vi "Page Sixe points.vi"() -> ()   [LabVIEW 2019]
uses:
  <userlib>/Exaprom PDF/Controls/Page Controls/Page size.ctl
  <userlib>/Exaprom PDF/Controls/Page Controls/Page Orientation.ctl
  C:/Program Files/National Instruments/LabVIEW 2019/user.lib/Exaprom PDF/DLL/itextsharp.dll
  DLL/itextsharp.dll
panel:
  out "Resulting page":T2
  in  "Page Size":cluster{"Width":sgl, "Height":sgl}
  in  "Orientation":T1
  out "Landscape":T3(array[cluster])
  out "Portrait":T3(array[cluster])
  out "Array":T4(array[cluster])
  in  "Page Size":T5=10 items=["Custom", "LETTER", "NOTE", "LEGAL", "TABLOID", "EXECUTIVE", "POSTCARD", "A0", "A1", "A2", "A3", "A4", "A5", "A6", "A7", "A8", "A9", "A10", "B0", "B1", "B2", "B3", "B4", "B5", "B6", "B7", "B8", "B9", "B10", "ARCH_E", "ARCH_D", "ARCH_C", "ARCH_B", "ARCH_A", "FLSA", "FLSE", "HALFLETTER", "_11X17", "ID_1", "ID_2", "ID_3", "LEDGER", "CROWN_QUARTO", "LARGE_CROWN_QUARTO", "DEMY_QUARTO", "ROYAL_QUARTO", "CROWN_OCTAVO", "LARGE_CROWN_OCTAVO", "DEMY_OCTAVO", "ROYAL_OCTAVO", "SMALL_PAPERBACK", "PENGUIN_SMALL_PAPERBACK", "PENGUIN_LARGE_PAPERBACK"]
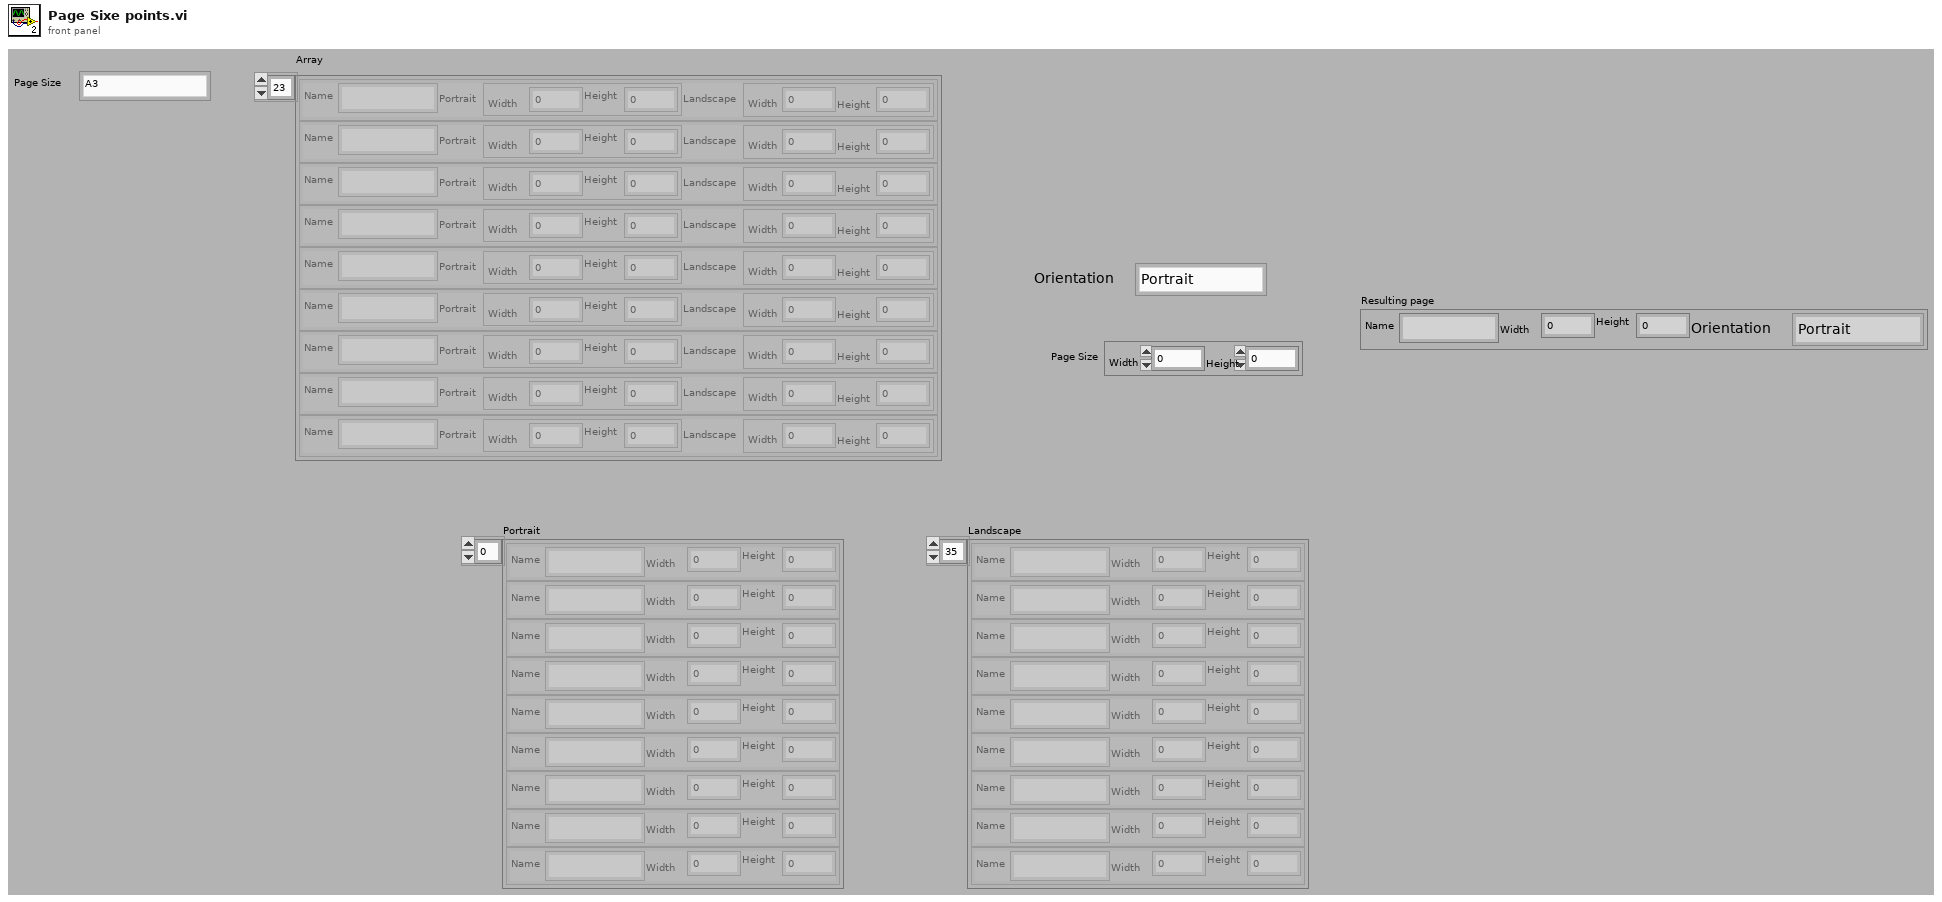
[diagram p1: front panel]
types:
  T1 = typedef "Page Orientation.ctl" = enum16{"Portrait", "Landscape"}
  T2 = cluster{"Name":string, "Width":sgl, "Height":sgl, "Orientation":T1}
  T3 = cluster{"Name":string, "Width":sgl, "Height":sgl}[]
  T4 = cluster{"Name":string, "Portrait":cluster{"Width":sgl, "Height":sgl}, "Landscape":cluster{"Width":sgl, "Height":sgl}}[]
  T5 = typedef "Page size.ctl" = i32
  T6 = cluster{string, cluster{"Width":sgl, "Height":sgl}, cluster{"Width":sgl, "Height":sgl}}
  T7 = cluster{"f":string, "Width":sgl, "Height":sgl, "Orientation":T1}
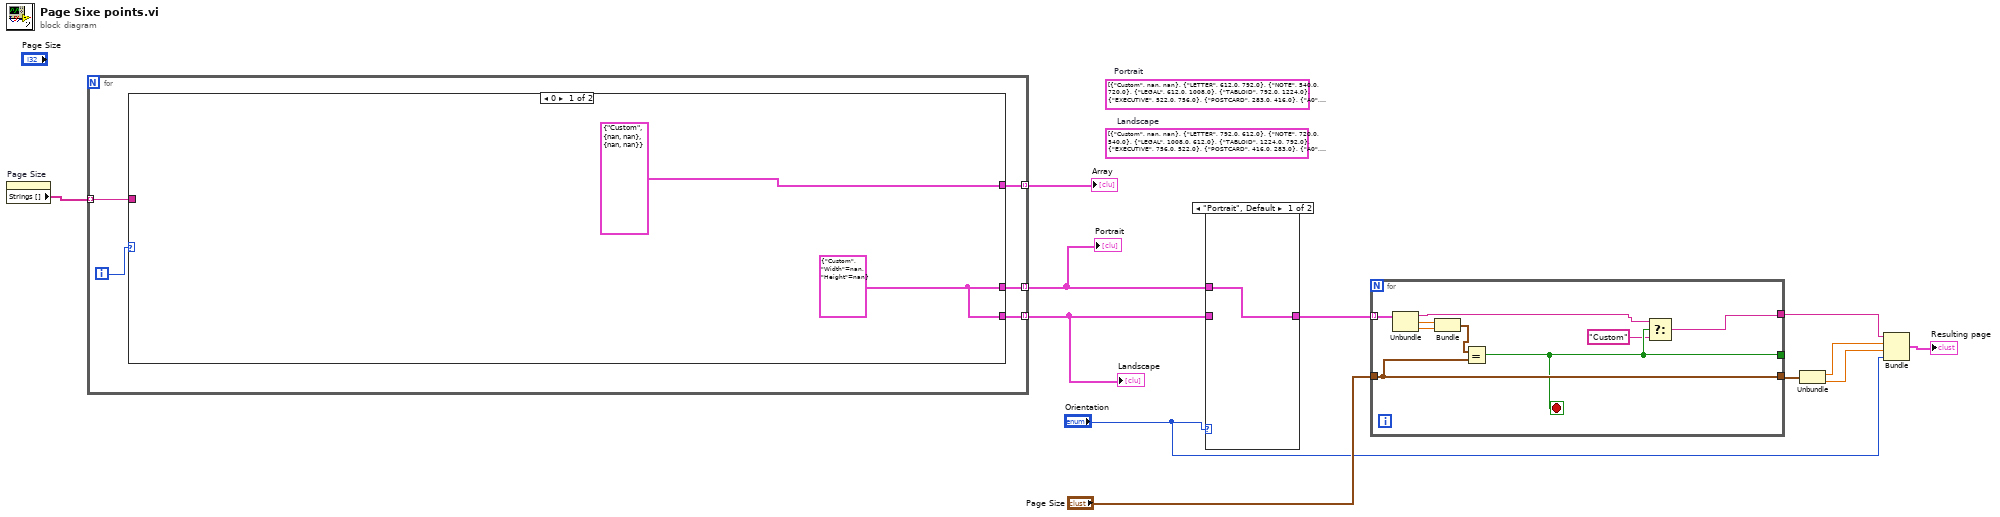
[diagram p0: block diagram]
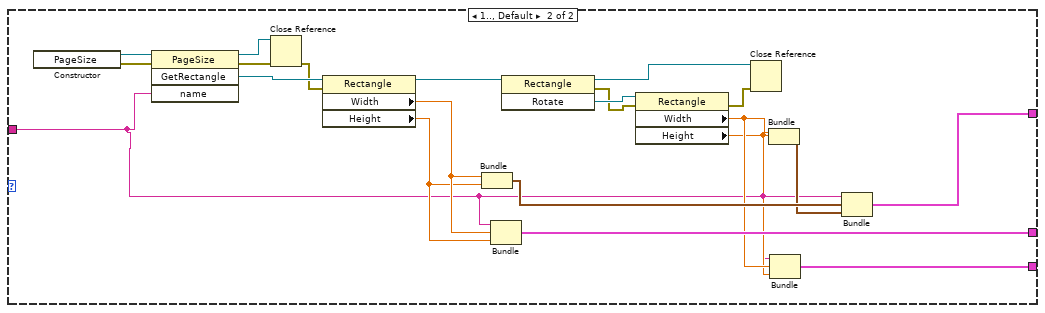
[diagram p3: hidden frame]
diagram:
  (unwired) T3 [{"Name"="Custom", "Width"=nan, "Height"=nan}, {"Name"="LETTER", "Width"=792.0, "Height"=612.0}, {"Name"="NOTE", "Width"=720.0, "Height"=540.0}, {"Name"="LEGAL", "Width"=1008.0, "Height"=612.0}, {"Name"="TABLOID", "Width"=1224.0, "Height"=792.0}, {"Name"="EXECUTIVE", "Width"=756.0, "Height"=522.0}, {"Name"="POSTCARD", "Width"=416.0, "Height"=283.0}, {"Name"="A0", "Width"=3370.0, "Height"=2384.0}, {"Name"="A1", "Width"=2384.0, "Height"=1684.0}, {"Name"="A2", "Width"=1684.0, "Height"=1191.0}, {"Name"="A3", "Width"=1191.0, "Height"=842.0}, {"Name"="A4", "Width"=842.0, "Height"=595.0}, {"Name"="A5", "Width"=595.0, "Height"=420.0}, {"Name"="A6", "Width"=420.0, "Height"=297.0}, {"Name"="A7", "Width"=297.0, "Height"=210.0}, {"Name"="A8", "Width"=210.0, "Height"=148.0}, {"Name"="A9", "Width"=148.0, "Height"=105.0}, {"Name"="A10", "Width"=105.0, "Height"=73.0}, {"Name"="B0", "Width"=4008.0, "Height"=2834.0}, {"Name"="B1", "Width"=2834.0, "Height"=2004.0}, {"Name"="B2", "Width"=2004.0, "Height"=1417.0}, {"Name"="B3", "Width"=1417.0, "Height"=1000.0}, {"Name"="B4", "Width"=1000.0, "Height"=708.0}, {"Name"="B5", "Width"=708.0, "Height"=498.0}, {"Name"="B6", "Width"=498.0, "Height"=354.0}, {"Name"="B7", "Width"=354.0, "Height"=249.0}, {"Name"="B8", "Width"=249.0, "Height"=175.0}, {"Name"="B9", "Width"=175.0, "Height"=124.0}, {"Name"="B10", "Width"=124.0, "Height"=87.0}, {"Name"="ARCH_E", "Width"=3456.0, "Height"=2592.0}, {"Name"="ARCH_D", "Width"=2592.0, "Height"=1728.0}, {"Name"="ARCH_C", "Width"=1728.0, "Height"=1296.0}, {"Name"="ARCH_B", "Width"=1296.0, "Height"=864.0}, {"Name"="ARCH_A", "Width"=864.0, "Height"=648.0}, {"Name"="FLSA", "Width"=936.0, "Height"=612.0}, {"Name"="FLSE", "Width"=936.0, "Height"=648.0}, {"Name"="HALFLETTER", "Width"=612.0, "Height"=396.0}, {"Name"="_11X17", "Width"=1224.0, "Height"=792.0}, {"Name"="ID_1", "Width"=153.0, "Height"=242.65}, {"Name"="ID_2", "Width"=210.0, "Height"=297.0}, {"Name"="ID_3", "Width"=249.0, "Height"=354.0}, {"Name"="LEDGER", "Width"=792.0, "Height"=1224.0}, {"Name"="CROWN_QUARTO", "Width"=697.0, "Height"=535.0}, {"Name"="LARGE_CROWN_QUARTO", "Width"=731.0, "Height"=569.0}, {"Name"="DEMY_QUARTO", "Width"=782.0, "Height"=620.0}, {"Name"="ROYAL_QUARTO", "Width"=884.0, "Height"=671.0}, {"Name"="CROWN_OCTAVO", "Width"=527.0, "Height"=348.0}, {"Name"="LARGE_CROWN_OCTAVO", "Width"=561.0, "Height"=365.0}, {"Name"="DEMY_OCTAVO", "Width"=612.0, "Height"=391.0}, {"Name"="ROYAL_OCTAVO", "Width"=663.0, "Height"=442.0}, {"Name"="SMALL_PAPERBACK", "Width"=504.0, "Height"=314.0}, {"Name"="PENGUIN_SMALL_PAPERBACK", "Width"=513.0, "Height"=314.0}, {"Name"="PENGUIN_LARGE_PAPERBACK", "Width"=561.0, "Height"=365.0}]  # Landscape
  (unwired) T3 [{"Name"="Custom", "Width"=nan, "Height"=nan}, {"Name"="LETTER", "Width"=612.0, "Height"=792.0}, {"Name"="NOTE", "Width"=540.0, "Height"=720.0}, {"Name"="LEGAL", "Width"=612.0, "Height"=1008.0}, {"Name"="TABLOID", "Width"=792.0, "Height"=1224.0}, {"Name"="EXECUTIVE", "Width"=522.0, "Height"=756.0}, {"Name"="POSTCARD", "Width"=283.0, "Height"=416.0}, {"Name"="A0", "Width"=2384.0, "Height"=3370.0}, {"Name"="A1", "Width"=1684.0, "Height"=2384.0}, {"Name"="A2", "Width"=1191.0, "Height"=1684.0}, {"Name"="A3", "Width"=842.0, "Height"=1191.0}, {"Name"="A4", "Width"=595.0, "Height"=842.0}, {"Name"="A5", "Width"=420.0, "Height"=595.0}, {"Name"="A6", "Width"=297.0, "Height"=420.0}, {"Name"="A7", "Width"=210.0, "Height"=297.0}, {"Name"="A8", "Width"=148.0, "Height"=210.0}, {"Name"="A9", "Width"=105.0, "Height"=148.0}, {"Name"="A10", "Width"=73.0, "Height"=105.0}, {"Name"="B0", "Width"=2834.0, "Height"=4008.0}, {"Name"="B1", "Width"=2004.0, "Height"=2834.0}, {"Name"="B2", "Width"=1417.0, "Height"=2004.0}, {"Name"="B3", "Width"=1000.0, "Height"=1417.0}, {"Name"="B4", "Width"=708.0, "Height"=1000.0}, {"Name"="B5", "Width"=498.0, "Height"=708.0}, {"Name"="B6", "Width"=354.0, "Height"=498.0}, {"Name"="B7", "Width"=249.0, "Height"=354.0}, {"Name"="B8", "Width"=175.0, "Height"=249.0}, {"Name"="B9", "Width"=124.0, "Height"=175.0}, {"Name"="B10", "Width"=87.0, "Height"=124.0}, {"Name"="ARCH_E", "Width"=2592.0, "Height"=3456.0}, {"Name"="ARCH_D", "Width"=1728.0, "Height"=2592.0}, {"Name"="ARCH_C", "Width"=1296.0, "Height"=1728.0}, {"Name"="ARCH_B", "Width"=864.0, "Height"=1296.0}, {"Name"="ARCH_A", "Width"=648.0, "Height"=864.0}, {"Name"="FLSA", "Width"=612.0, "Height"=936.0}, {"Name"="FLSE", "Width"=648.0, "Height"=936.0}, {"Name"="HALFLETTER", "Width"=396.0, "Height"=612.0}, {"Name"="_11X17", "Width"=792.0, "Height"=1224.0}, {"Name"="ID_1", "Width"=242.65, "Height"=153.0}, {"Name"="ID_2", "Width"=297.0, "Height"=210.0}, {"Name"="ID_3", "Width"=354.0, "Height"=249.0}, {"Name"="LEDGER", "Width"=1224.0, "Height"=792.0}, {"Name"="CROWN_QUARTO", "Width"=535.0, "Height"=697.0}, {"Name"="LARGE_CROWN_QUARTO", "Width"=569.0, "Height"=731.0}, {"Name"="DEMY_QUARTO", "Width"=620.0, "Height"=782.0}, {"Name"="ROYAL_QUARTO", "Width"=671.0, "Height"=884.0}, {"Name"="CROWN_OCTAVO", "Width"=348.0, "Height"=527.0}, {"Name"="LARGE_CROWN_OCTAVO", "Width"=365.0, "Height"=561.0}, {"Name"="DEMY_OCTAVO", "Width"=391.0, "Height"=612.0}, {"Name"="ROYAL_OCTAVO", "Width"=442.0, "Height"=663.0}, {"Name"="SMALL_PAPERBACK", "Width"=314.0, "Height"=504.0}, {"Name"="PENGUIN_SMALL_PAPERBACK", "Width"=314.0, "Height"=513.0}, {"Name"="PENGUIN_LARGE_PAPERBACK", "Width"=365.0, "Height"=561.0}]  # Portrait
  n1 = property on="Page Size" class="Ring (strict)"() -> ("Strings []"=w12:string[])  [unwired: 2 in, 2 out]
  n2 = for {
    tunnel: w12 -> [w17] mode=indexing
    tunnel: [w15] -> w11 mode=indexing
    tunnel: [w14] -> w9 mode=indexing
    tunnel: [w13] -> w10 mode=indexing
    i -> [w16]
    n3 = case shown="0" w16 {
      tunnel: w17 -> [_ w21]
      tunnel: [T6 {"Custom", {"Width"=nan, "Height"=nan}, {"Width"=nan, "Height"=nan}} w27] -> w15
      tunnel: [w18 w24] -> w14
      tunnel: [w18 w20] -> w13
      frame 0 {
        w18 = cluster{string, "Width":sgl, "Height":sgl} {"Custom", "Width"=nan, "Height"=nan}
      }
      frame 1.., Default {
        n4 = constructor class="PageSize"() -> (reference out=w40:refnum<k24>, error out=w39:errorcluster)  [unwired: 3 in, 1 out]
        n5 = invoke class="PageSize" method="GetRectangle"(reference=w40, error in=w39, "name"=w21) -> (reference out=w37:refnum<k24>, error out=w38:errorcluster, "GetRectangle"=w36:refnum<k24>)  [unwired: 1 in, 1 out]
        n6 = Close Reference(reference=w37, error in (no error)=w38) -> (error out=w35:errorcluster)
        n7 = property class="Rectangle"(reference=w36, error in=w35) -> (reference out=w33:refnum<k24>, "Width"=w26:sgl, "Height"=w25:sgl)  [unwired: 1 out]
        n8 = Bundle("Width"=w26, "Height"=w25) -> (w29:cluster{"Width":sgl, "Height":sgl})  [unwired: 1 in]
        n9 = Bundle(w21, "Width"=w26, "Height"=w25) -> (w24:cluster{string, "Width":sgl, "Height":sgl})  [unwired: 1 in]
        n10 = invoke class="Rectangle" method="Rotate"(reference=w33) -> (reference out=w34:refnum<k24>, error out=w30:errorcluster, "Rotate"=w31:refnum<k24>)  [unwired: 2 in]
        n11 = property class="Rectangle"(reference=w31, error in=w30) -> (error out=w32:errorcluster, "Width"=w23:sgl, "Height"=w22:sgl)  [unwired: 1 out]
        n12 = Close Reference(reference=w34, error in (no error)=w32) -> ()  [unwired: 1 out]
        n13 = Bundle("Width"=w23, "Height"=w22) -> (w28:cluster{"Width":sgl, "Height":sgl})  [unwired: 1 in]
        n14 = Bundle(w21, "Width"=w23, "Height"=w22) -> (w20:cluster{string, "Width":sgl, "Height":sgl})  [unwired: 1 in]
        n15 = Bundle(w21, w29, w28) -> (w27:T6)  [unwired: 1 in]
      }
    }
  }
  "Array" <- w11
  "Portrait" <- w9
  "Landscape" <- w10
  n16 = case shown="\"Portrait\", Default" "Orientation" {
    tunnel: [w41 w42] -> w8
    tunnel: w10 -> [_ w42]
    tunnel: w9 -> [w41 _]
    frame "Portrait", Default {
    }
    frame "Landscape" {
    }
  }
  n17 = for {
    tunnel: w8 -> [w51] mode=indexing
    tunnel: "Page Size" -> [w47]
    tunnel: [w43] -> w6
    tunnel: [w47] -> w5
    tunnel: [w46] -> _
    stop <- w46 stop-if-true
    n18 = Unbundle(w51) -> (w44:string, "Width"=w50:sgl, "Height"=w49:sgl)
    n19 = Bundle("Width"=w50, "Height"=w49) -> (w48:cluster{"Width":sgl, "Height":sgl})  [unwired: 1 in]
    n20 = Equal?(x=w48, y=w47) -> (x = y?=w46:bool)
    n21 = Select(t=w44, s=w46, f="Custom") -> (s? t:f=w43:string)
  }
  n22 = Unbundle(w5) -> ("Width"=w4:sgl, "Height"=w3:sgl)
  n23 = Bundle("f"=w6, "Width"=w4, "Height"=w3, "Orientation"="Orientation") -> (→"Resulting page":T7)  [unwired: 1 in]
